vi "Array to Tag.vi"(8 "error in (no error)":T1, 11 "1D array":string[](array[string])) -> (0 "error out":T1, 3 "Array":T2[](array[typedef]))   [LabVIEW 2018]
uses:
  CTL/Tags.ctl
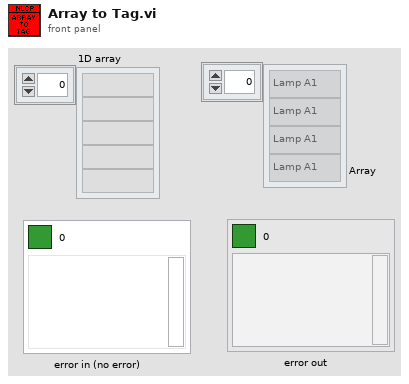
[diagram p1: front panel]
types:
  T1 = cluster{"Boolean Round":bool, "code":i32, "source":string}
  T2 = typedef "Tags.ctl" = enum16{"Lamp A1", "Lamp B1", "Lamp C1", "Lamp D1", "Lamp E1", "Lamp F1", "Lamp G1", "Lamp H1", "Lamp A2", "Lamp B2", "Lamp C2", "Lamp D2", "Lamp E2", "Lamp F2", "Lamp G2", "Lamp H2", "Ack A1", "Ack B1", "Ack C1", "Ack D1", "Ack E1", "Ack F1", "Ack G1", "Ack H1", "Ack A2", "Ack B2", "Ack C2", "Ack D2", "Ack E2", "Ack F2", "Ack G2", "Ack H2", "SSM", "SAS", "LSM", ""}
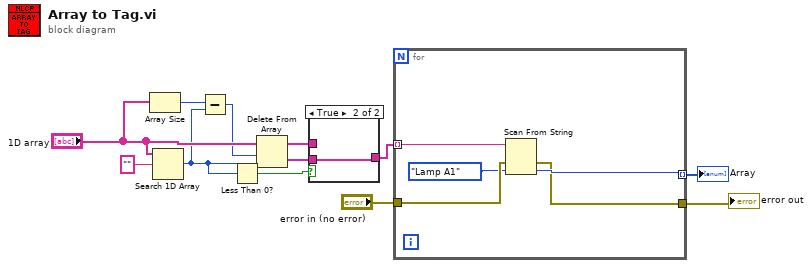
[diagram p0: block diagram]
diagram:
  n1 = Array Size(array="1D array") -> (size(s)=w10:i32)
  n2 = Search 1D Array(1D array="1D array", element="") -> (index of element=w5:i32)  [unwired: 1 in]
  n3 = Subtract(x=w10, y=w5) -> (x-y=w6:i32)
  n4 = Less Than 0?(x=w5) -> (x < 0?=w4:bool)
  n5 = Delete From Array(array="1D array", length=w6, index=w5) -> (deleted portion=w3:string[], array with subset deleted=w1:string[])
  n6 = case shown="True" w4 {
    tunnel: [w13 w14] -> w2
    tunnel: w3 -> [_ w14]
    tunnel: w1 -> [w13 _]
    frame False {
    }
    frame True {
    }
  }
  n7 = for {
    tunnel: [w19] -> w11 mode=indexing
    tunnel: "error in (no error)" -> [w18]
    tunnel: [w17] -> w8
    tunnel: w2 -> [w15] mode=indexing
    n8 = Scan From String(input string=w15, error in=w18, default 1=Tags."Lamp A1" ("Tag")) -> (error out=w17:errorcluster, output 1=w19:T2)  [unwired: 2 in, 2 out]
  }
  "Array" <- w11
  "error out" <- w8
